vi "test.vi"() -> ()   [LabVIEW 2015]
panel:
  in  "布尔":bool
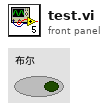
[diagram p1: front panel]
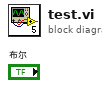
[diagram p0: block diagram]
diagram:
